vi "replay logger_coMD.vi"(8 "Error in":errorcluster) -> (0 "Error out":errorcluster)   [LabVIEW 2012]
uses:
  <vilib>/Utility/VariantDataType/Type.ctl
  CommonResource VIs/Variant_to_X/Variant_to_Enum_U8.vi
  <vilib>/Utility/file.llb/Write To Spreadsheet File (string).vi
  CommonResource VIs/Variant_to_X/Variant_to_I8.vi
  CommonResource VIs/Variant_to_X/Variant_to_I16.vi
  CommonResource VIs/Variant_to_X/Variant_to_I32.vi
  CommonResource VIs/Variant_to_X/Variant_to_I64.vi
  CommonResource VIs/Variant_to_X/Variant_to_U8.vi
  CommonResource VIs/Variant_to_X/Variant_to_U16.vi
  CommonResource VIs/Variant_to_X/Variant_to_U32.vi
  CommonResource VIs/Variant_to_X/Variant_to_U64.vi
  CommonResource VIs/Variant_to_X/Variant_to_SGL.vi
  CommonResource VIs/Variant_to_X/Variant_to_DBL.vi
  CommonResource VIs/Variant_to_X/Variant_to_EXT.vi
  CommonResource VIs/Variant_to_X/Variant_to_CSG.vi
  CommonResource VIs/Variant_to_X/Variant_to_CDB.vi
  CommonResource VIs/Variant_to_X/Variant_to_CXT.vi
  CommonResource VIs/Variant_to_X/Variant_to_Enum_U16.vi
  CommonResource VIs/Variant_to_X/Variant_to_Enum_U32.vi
  CommonResource VIs/Variant_to_X/Variant_to_Enum_U64.vi
  CommonResource VIs/Variant_to_X/Variant_to_Boolean.vi
  CommonResource VIs/Variant_to_X/Variant_to_String.vi
  CommonResource VIs/Variant_to_X/Variant_to_Path.vi
  CommonResource VIs/Variant_to_X/Variant_to_Array.vi
  CommonResource VIs/Variant_to_X/Variant_to_Cluster.vi
  CommonResource VIs/Variant_to_X/Variant_to_Waveform_info.vi
  CommonResource VIs/Variant_to_X/Variant_to_Timestamp.vi
  CommonResource VIs/Variant_to_X/Variant_to_Refnum.vi
  CommonResource VIs/Variant_to_X/Variant_to_Fixed_point.vi
  <vilib>/Utility/VariantDataType/VariantType.lvlib
  CommonResource VIs/Variant_to_X/Variant_to_Waveform.vi
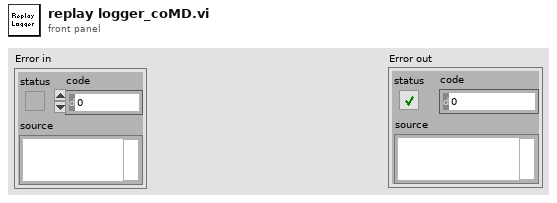
[diagram p1: front panel]
types:
  T1 = typedef "VariantType.lvlib/Type.ctl" = enum8{"Invalid Type", "Void", "I8", "I16", "I32", "I64", "U8", "U16", "U32", "U64", "Single Float", "Double Float", "Extended Float", "Single Complex", "Double Complex", "Extended Complex", "Enum U8", "Enum U16", "Enum U32", "Enum U64", "Single Float With Unit", "Double Float With Unit", "Extended Float With Unit", "Single Complex with Unit", "Double Complex with Unit", "Extended Complex with Unit", "Boolean", "String", "Path", "Picture", "Tag", "Array", "Cluster", "Variant", "LV Variant", "Waveform", "Timestamp", "Digital Waveform", "Digital Data", "ExpressData", "Refnum", "External Data", "VI", "Poly VI", "LabVIEW Class Instance", "Fixed Point"}
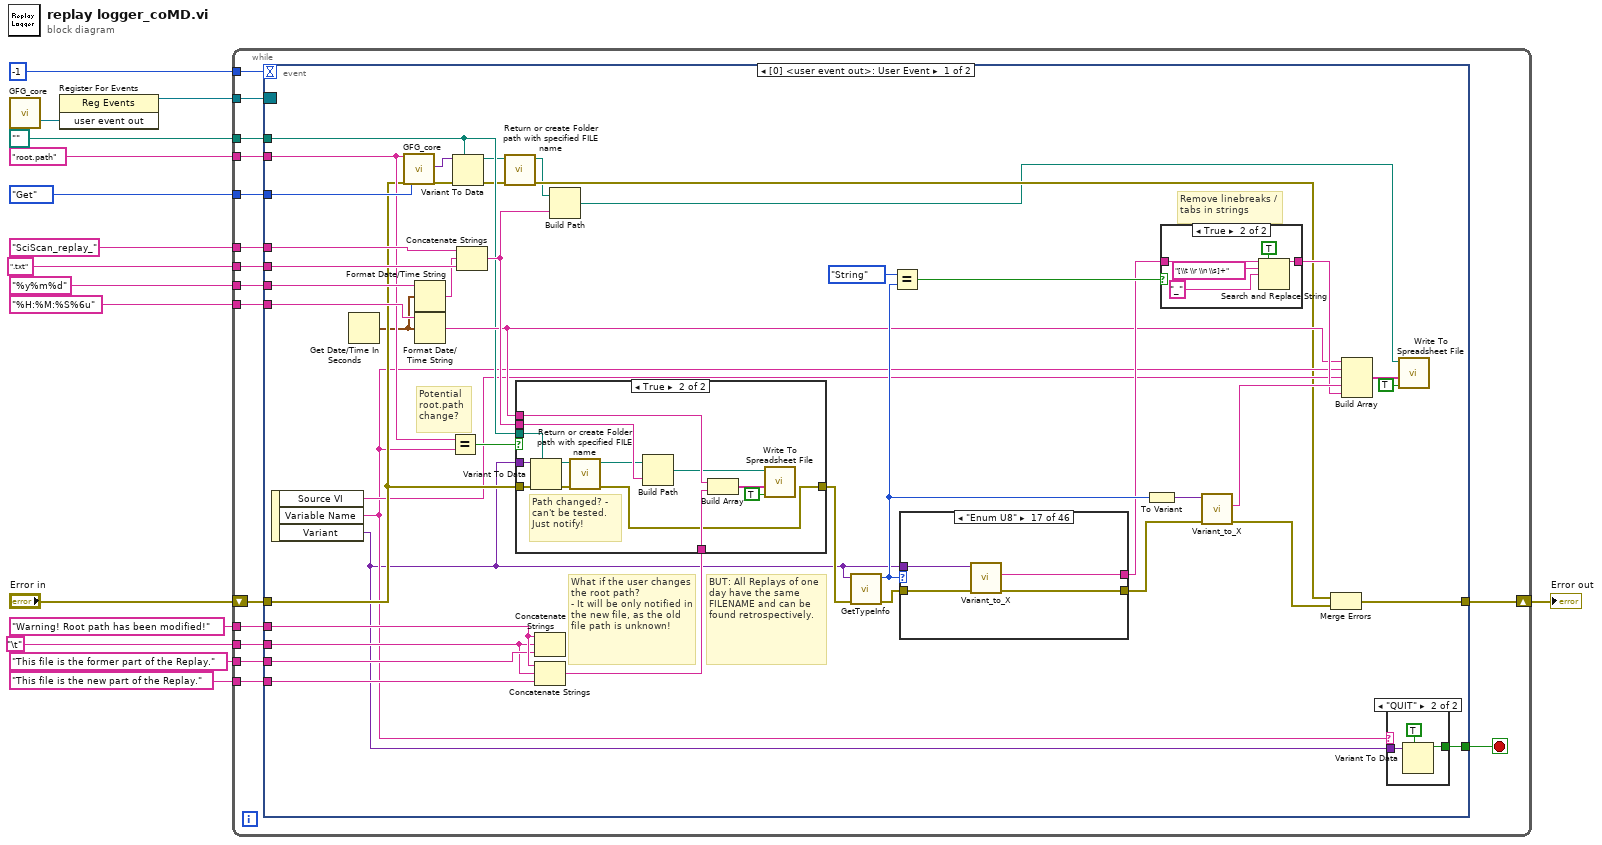
[diagram p0: block diagram]
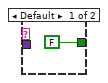
[diagram p2: hidden frame]
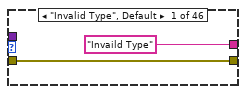
[diagram p5: hidden frame]
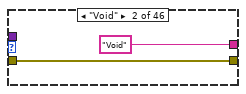
[diagram p6: hidden frame]
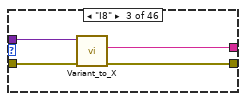
[diagram p7: hidden frame]
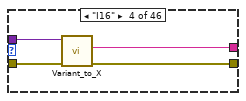
[diagram p8: hidden frame]
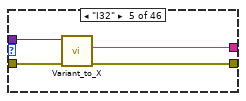
[diagram p9: hidden frame]
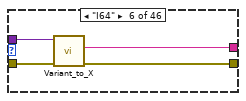
[diagram p10: hidden frame]
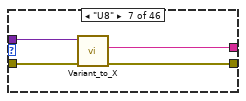
[diagram p11: hidden frame]
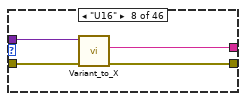
[diagram p12: hidden frame]
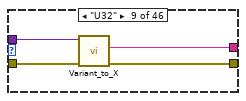
[diagram p13: hidden frame]
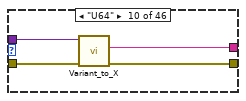
[diagram p14: hidden frame]
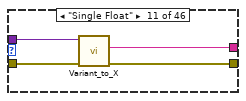
[diagram p15: hidden frame]
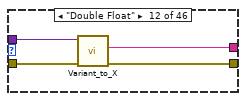
[diagram p16: hidden frame]
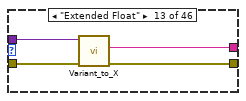
[diagram p17: hidden frame]
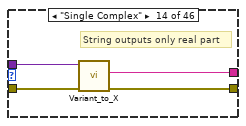
[diagram p18: hidden frame]
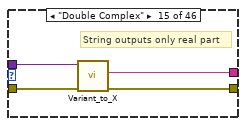
[diagram p19: hidden frame]
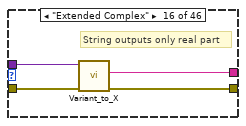
[diagram p20: hidden frame]
diagram:
  n1 = call "GFG_core.vi"() -> ("user event out"=w4:refnum<user-event>)  [unwired: 13 in, 6 out]
  n2 = register-events(w4) -> (reference out=w3:refnum<event-registration>)  [unwired: 2 in, 1 out]
  n3 = while {
    tunnel: "SciScan_replay_" -> [w32]
    tunnel: ".txt" -> [w31]
    tunnel: "%y%m%d" -> [w30]
    tunnel: enum16{"Init", "Set", "Get", "Clear"}."Get" ("Action") -> [w29]
    tunnel: "%H:%M:%S%6u" -> [w28]
    tunnel: "root.path" ("Variable Name in") -> [w27]
    tunnel: "Warning! Root path has been modified!" -> [w25]
    tunnel: "This file is the former part of the Replay." -> [w24]
    tunnel: "This file is the new part of the Replay." -> [w23]
    tunnel: path "" -> [w22]
    tunnel: "\t" -> [w21]
    tunnel: w3 -> [w20]
    shift-right: [w19] -> w2
    shift-left: "Error in" -> [w26]
    tunnel: -1 -> [w18]
    stop <- w17 stop-if-true
    n4 = event shown="[0] <user event out>: User Event" {
      selector: w20 -> [_ _]
      dyn-events: _ -> [_ _]
      timeout: w18 -> [_ _]
      tunnel: w32 -> [w75 _]
      tunnel: w31 -> [w74 _]
      tunnel: [w73 w255] -> w19
      tunnel: w30 -> [w72 _]
      tunnel: w29 -> [w68 _]
      tunnel: w28 -> [w61 _]
      tunnel: w27 -> [w54 _]
      tunnel: w26 -> [w52 w255]
      tunnel: w25 -> [w49 _]
      tunnel: w24 -> [w48 _]
      tunnel: w23 -> [w47 _]
      tunnel: w22 -> [w44 _]
      tunnel: w21 -> [w43 _]
      tunnel: [w39 FALSE] -> w17
      event User Event {
        # "BUT: All Replays of one day have the same FILENAME and can be found retrospectively."
        # "Potential root.path change?"
        # "Remove linebreaks / tabs in strings"
        # "What if the user changes the root path?\n- It will be only notified in the new file, as the old file path is unknown!"
        n5 = event-data() -> ("Source VI"=w42:string, "Variable Name"=w41:string, "Variant"=w40:variant)  [unwired: 1 in]
        n6 = Get Date/Time In Seconds() -> (seconds since 1Jan1904=w38:timestamp)
        n7 = call "GFG_core.vi"("Variable Name in"=w54, "error in (no error)"=w52, "Action"=w68) -> ("Variant Out"=w67:variant, "error out"=w66:errorcluster)  [unwired: 10 in, 5 out]
        n8 = Format Date/Time String(time format string (%c)=w72, seconds (now)=w38) -> (date/time string=w69:string)  [unwired: 1 in]
        n9 = Format Date/Time String(time format string (%c)=w61, seconds (now)=w38) -> (date/time string=w45:string)  [unwired: 1 in]
        n10 = Equal?(x=w54, y=w41) -> (x = y?=w53:bool)
        n11 = Variant To Data(error in=w66, type=w44, Variant=w67) -> (data=w34:path, error out=w37:errorcluster)
        n12 = Concatenate Strings(w75, w69, w74) -> (w50:string)
        n13 = call "Return or create Folder path with specified FILE name.vi"("error in (no error)"=w37, "File Path IN"=w34) -> ("error out"=w36:errorcluster, "Folder Path OUT"=w33:path)  [unwired: 8 in]
        n14 = Concatenate Strings(w49, w43, w48) -> ()  [unwired: 1 out]
        n15 = Concatenate Strings(w49, w43, w47) -> (w46:string)
        n16 = case shown="True" w53 {
          tunnel: w44 -> [_ w91]
          tunnel: w40 -> [_ w93]
          tunnel: w52 -> [w80 w92]
          tunnel: [w80 w82] -> w51
          tunnel: w50 -> [_ w90]
          tunnel: w46 -> [_ w89]
          tunnel: w45 -> [_ w88]
          frame False {
          }
          frame True {
            # "Path changed? - can't be tested. Just notify!"
            n17 = Variant To Data(error in=w92, type=w91, Variant=w93) -> (data=w84:path, error out=w83:errorcluster)
            n18 = call "Return or create Folder path with specified FILE name.vi"("error in (no error)"=w83, "File Path IN"=w84) -> ("error out"=w82:errorcluster, "Folder Path OUT"=w81:path)  [unwired: 8 in]
            n19 = Build Path(base path=w81, name or relative path=w90) -> (appended path=w86:path)
            n20 = Build Array(w88, w89) -> (w85:string[])
            n21 = call-poly <vilib>:"Write To Spreadsheet File.vi"("append to file? (new file:F)"=TRUE, "1D data"=w85, "file path (dialog if empty)"=w86) -> ()  [unwired: 5 in, 1 out]
          }
        }
        n22 = Build Path(base path=w33, name or relative path=w50) -> (appended path=w35:path)
        n23 = call <vilib>:"GetTypeInfo.vi"("error in (no error)"=w51, "Variant"=w40) -> ("error out"=w65:errorcluster, "Type Enum"=w59:T1)  [unwired: 5 in, 3 out]
        n24 = Equal?(x=Type."String" ("Type Enum"), y=w59) -> (x = y?=w57:bool)
        n25 = case shown="\"Enum U8\"" w59 {
          tunnel: ["Invaild Type" "Void" w105 w108 w112 w116 w120 w124 w128 w133 w137 w140 w144 w148 w152 w156 w160 w165 w168 w172 "{Single Float With Unit}" "{Double Float With Unit}" "{Extended Float With Unit}" "{Single Complex with Unit}" "{Double Complex with Unit}" "{Extended Complex with Unit}" w188 w192 w196 "{Picture}" "{Tag}" w204 w208 "{Variant}" "{LV Variant}" w216 w228 "{Digital Wavefrom}" "{Digital Data}" "{ExpressData}" w238 "{External Data}" "{VI}" "{Poly VI}" "{LabVIEW Class Instance}" w250] -> w56
          tunnel: w40 -> [_ _ w107 w111 w115 w119 w123 w127 w131 w135 w139 w141 w147 w151 w155 w157 w163 w167 w171 w175 _ _ _ _ _ _ w191 w195 w199 _ _ w205 w211 _ _ w219 w231 _ _ _ w241 _ _ _ _ w253]
          tunnel: w65 -> [w100 w102 w106 w110 w114 w118 w122 w126 w130 w134 w138 w143 w146 w150 w154 w159 w162 w166 w170 w174 w177 w179 w181 w183 w185 w187 w190 w194 w198 w201 w203 w207 w210 w213 w215 w218 w230 w232 w235 w237 w240 w243 w245 w247 w249 w252]
          tunnel: [w100 w102 w104 w109 w113 w117 w121 w125 w129 w132 w136 w142 w145 w149 w153 w158 w161 w164 w169 w173 w177 w179 w181 w183 w185 w187 w189 w193 w197 w201 w203 w206 w209 w213 w215 w217 w229 w232 w235 w237 w239 w243 w245 w247 w249 w251] -> w63
          frame "Invalid Type", Default {
          }
          frame "Void" {
          }
          frame "I8" {
            n26 = call-poly "Variant_to_X.vi"("Error in"=w106, "Value (in)"=w107) -> ("Error out"=w104:errorcluster, "Value (string)"=w105:string)  [unwired: 7 in, 1 out]
          }
          frame "I16" {
            n27 = call-poly "Variant_to_X.vi"("Error in"=w110, "Value (in)"=w111) -> ("Error out"=w109:errorcluster, "Value (string)"=w108:string)  [unwired: 7 in, 1 out]
          }
          frame "I32" {
            n28 = call-poly "Variant_to_X.vi"("Error in"=w114, "Value (in)"=w115) -> ("Error out"=w113:errorcluster, "Value (string)"=w112:string)  [unwired: 7 in, 1 out]
          }
          frame "I64" {
            n29 = call-poly "Variant_to_X.vi"("Error in"=w118, "Value (in)"=w119) -> ("Error out"=w117:errorcluster, "Value (string)"=w116:string)  [unwired: 7 in, 1 out]
          }
          frame "U8" {
            n30 = call-poly "Variant_to_X.vi"("Error in"=w122, "Value (in)"=w123) -> ("Error out"=w121:errorcluster, "Value (string)"=w120:string)  [unwired: 7 in, 1 out]
          }
          frame "U16" {
            n31 = call-poly "Variant_to_X.vi"("Error in"=w126, "Value (in)"=w127) -> ("Error out"=w125:errorcluster, "Value (string)"=w124:string)  [unwired: 7 in, 1 out]
          }
          frame "U32" {
            n32 = call-poly "Variant_to_X.vi"("Error in"=w130, "Value (in)"=w131) -> ("Error out"=w129:errorcluster, "Value (string)"=w128:string)  [unwired: 7 in, 1 out]
          }
          frame "U64" {
            n33 = call-poly "Variant_to_X.vi"("Error in"=w134, "Value (in)"=w135) -> ("Error out"=w132:errorcluster, "Value (string)"=w133:string)  [unwired: 7 in, 1 out]
          }
          frame "Single Float" {
            n34 = call-poly "Variant_to_X.vi"("Error in"=w138, "Value (in)"=w139) -> ("Error out"=w136:errorcluster, "Value (string)"=w137:string)  [unwired: 7 in, 1 out]
          }
          frame "Double Float" {
            n35 = call-poly "Variant_to_X.vi"("Error in"=w143, "Value (in)"=w141) -> ("Error out"=w142:errorcluster, "Value (string)"=w140:string)  [unwired: 7 in, 1 out]
          }
          frame "Extended Float" {
            n36 = call-poly "Variant_to_X.vi"("Error in"=w146, "Value (in)"=w147) -> ("Error out"=w145:errorcluster, "Value (string)"=w144:string)  [unwired: 7 in, 1 out]
          }
          frame "Single Complex" {
            # "String outputs only real part"
            n37 = call-poly "Variant_to_X.vi"("Error in"=w150, "Value (in)"=w151) -> ("Error out"=w149:errorcluster, "Value (string)"=w148:string)  [unwired: 7 in, 1 out]
          }
          frame "Double Complex" {
            # "String outputs only real part"
            n38 = call-poly "Variant_to_X.vi"("Error in"=w154, "Value (in)"=w155) -> ("Error out"=w153:errorcluster, "Value (string)"=w152:string)  [unwired: 7 in, 1 out]
          }
          frame "Extended Complex" {
            # "String outputs only real part"
            n39 = call-poly "Variant_to_X.vi"("Error in"=w159, "Value (in)"=w157) -> ("Error out"=w158:errorcluster, "Value (string)"=w156:string)  [unwired: 7 in, 1 out]
          }
          frame "Enum U8" {
            n40 = call-poly "Variant_to_X.vi"("Error in"=w162, "Value (in)"=w163) -> ("Error out"=w161:errorcluster, "Value (string)"=w160:string)  [unwired: 7 in, 1 out]
          }
          frame "Enum U16" {
            n41 = call-poly "Variant_to_X.vi"("Error in"=w166, "Value (in)"=w167) -> ("Error out"=w164:errorcluster, "Value (string)"=w165:string)  [unwired: 7 in, 1 out]
          }
          frame "Enum U32" {
            n42 = call-poly "Variant_to_X.vi"("Error in"=w170, "Value (in)"=w171) -> ("Error out"=w169:errorcluster, "Value (string)"=w168:string)  [unwired: 7 in, 1 out]
          }
          frame "Enum U64" {
            n43 = call-poly "Variant_to_X.vi"("Error in"=w174, "Value (in)"=w175) -> ("Error out"=w173:errorcluster, "Value (string)"=w172:string)  [unwired: 7 in, 1 out]
          }
          frame "Single Float With Unit" {
          }
          frame "Double Float With Unit" {
          }
          frame "Extended Float With Unit" {
          }
          frame "Single Complex with Unit" {
          }
          frame "Double Complex with Unit" {
          }
          frame "Extended Complex with Unit" {
          }
          frame "Boolean" {
            n44 = call-poly "Variant_to_X.vi"("Error in"=w190, "Value (in)"=w191) -> ("Error out"=w189:errorcluster, "Value (string)"=w188:string)  [unwired: 7 in, 1 out]
          }
          frame "String" {
            n45 = call-poly "Variant_to_X.vi"("Error in"=w194, "Value (in)"=w195) -> ("Error out"=w193:errorcluster, "Value (string)"=w192:string)  [unwired: 7 in, 1 out]
          }
          frame "Path" {
            n46 = call-poly "Variant_to_X.vi"("Error in"=w198, "Value (in)"=w199) -> ("Error out"=w197:errorcluster, "Value (string)"=w196:string)  [unwired: 7 in, 1 out]
          }
          frame "Picture" {
          }
          frame "Tag" {
          }
          frame "Array" {
            n47 = call-poly "Variant_to_X.vi"("Error in"=w207, "Value (in)"=w205) -> ("Error out"=w206:errorcluster, "Value (string)"=w204:string)  [unwired: 7 in, 1 out]
          }
          frame "Cluster" {
            n48 = call-poly "Variant_to_X.vi"("Error in"=w210, "Value (in)"=w211) -> ("Error out"=w209:errorcluster, "Value (string)"=w208:string)  [unwired: 7 in, 1 out]
          }
          frame "Variant" {
          }
          frame "LV Variant" {
          }
          frame "Waveform" {
            n49 = disable-structure shown="Enabled" {
              disable-tunnel: w219 -> [w223 w227]
              disable-tunnel: w218 -> [w222 w226]
              disable-tunnel: [w221 w225] -> w217
              disable-tunnel: [w220 w224] -> w216
              frame Disabled {
                n50 = call-poly "Variant_to_X.vi"("Error in"=w222, "Value (in)"=w223) -> ("Error out"=w221:errorcluster, "Value (string)"=w220:string)  [unwired: 7 in, 1 out]
              }
              frame Enabled {
                n51 = call-poly "Variant_to_X.vi"("Error in"=w226, "Value (in)"=w227) -> ("Error out"=w225:errorcluster, "Value (string)"=w224:string)  [unwired: 7 in, 1 out]
              }
            }
          }
          frame "Timestamp" {
            n52 = call-poly "Variant_to_X.vi"("Error in"=w230, "Value (in)"=w231) -> ("Error out"=w229:errorcluster, "Value (string)"=w228:string)  [unwired: 7 in, 1 out]
          }
          frame "Digital Waveform" {
          }
          frame "Digital Data" {
          }
          frame "ExpressData" {
          }
          frame "Refnum" {
            n53 = call-poly "Variant_to_X.vi"("Error in"=w240, "Value (in)"=w241) -> ("Error out"=w239:errorcluster, "Value (string)"=w238:string)  [unwired: 5 in, 3 out]
          }
          frame "External Data" {
          }
          frame "VI" {
          }
          frame "Poly VI" {
          }
          frame "LabVIEW Class Instance" {
          }
          frame "Fixed Point" {
            n54 = call-poly "Variant_to_X.vi"("Error in"=w252, "Value (in)"=w253) -> ("Error out"=w251:errorcluster, "Value (string)"=w250:string)  [unwired: 7 in, 1 out]
          }
        }
        n55 = To Variant(anything=w59) -> (Variant=w64:variant)
        n56 = case shown="True" w57 {
          tunnel: w56 -> [w94 w96]
          tunnel: [w94 w95] -> w55
          frame False {
          }
          frame True {
            n57 = Search and Replace String(replace all?=TRUE ("replace all? (F)"), input string=w96, search string="[\\t \\r \\n \\s]+", replace string="_" ("replace string (\"\")")) -> (result string=w95:string)  [unwired: 4 in, 3 out]
          }
        }
        n58 = call-poly "Variant_to_X.vi"("Error in"=w63, "Value (in)"=w64) -> ("Error out"=w62:errorcluster, "Value (string)"=w60:string)  [unwired: 7 in, 1 out]
        n59 = Merge Errors(w36, w62) -> (w73:errorcluster)
        n60 = Build Array(w45, w41, w42, w60, w55) -> (w71:string[])
        n61 = case shown="\"QUIT\"" w41 {
          tunnel: [FALSE w77] -> w39
          tunnel: w40 -> [_ w79]
          frame Default {
          }
          frame "QUIT" {
            n62 = Variant To Data(type=TRUE, Variant=w79) -> (data=w77:bool)  [unwired: 1 in, 1 out]
          }
        }
        n63 = call-poly <vilib>:"Write To Spreadsheet File.vi"("append to file? (new file:F)"=TRUE, "1D data"=w71, "file path (dialog if empty)"=w35) -> ()  [unwired: 5 in, 1 out]
      }
      event Timeout {
        n64 = event-data() -> ()  [unwired: 1 in, 1 out]
      }
    }
  }
  "Error out" <- w2
